vi "Begin.vi"(8 "error in":errorcluster) -> (0 "error out":errorcluster)   [LabVIEW 2020]
doc: "Called before other user functions, this VI is expected to open initial I/O refnums, load in file data, and do all program initialization. Notice that the <B>error out</B> terminal is simply used for data flow. Wiring it to other structures or subVIs ensures that this VI runs first."
uses:
  <vilib>/Rock Robotics/WPI/SafetyOutput/WPI_SafetyOutputConfigMenu.ctl
  <vilib>/Rock Robotics/WPI/DriverStation/WPI_DriverStationRobotMode2.ctl
  <vilib>/Rock Robotics/WPI/Joystick/WPI_JoystickDeviceEnum.ctl
  <vilib>/Rock Robotics/WPI/Solenoid/WPI_SolenoidChannel.ctl
  <vilib>/Rock Robotics/WPI/ThirdParty/REV Robotics/REVLib/Typedef/Spark MAX Idle Mode.ctl
  <vilib>/Rock Robotics/WPI/ThirdParty/Phoenix-LabVIEW/Motor Controller/Controls/CTRE_Phoenix_MotorControl_NeutralMode.ctl
  Robot Global Data.vi
  <vilib>/Rock Robotics/Network Tables/NT Write String Array.vi
  <vilib>/Rock Robotics/WPI/Solenoid/WPI_SolenoidOpenDouble.vi
  <vilib>/Rock Robotics/WPI/RobotDrive/WPI_RobotDriveOpen2MotorWithExistingMotors.vi
  <vilib>/Rock Robotics/WPI/Utilities/WPI_GetSetVariantRefNum.vi
  <vilib>/Rock Robotics/SystemInterfaces/AI/FPGA_AIChannel.ctl
  <vilib>/Rock Robotics/SystemInterfaces/DIO/FPGA_DIOChannel.ctl
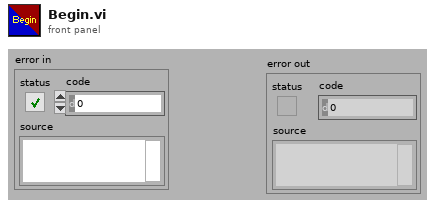
[diagram p1: front panel]
types:
  T1 = typedef "FPGA_DIOChannel.ctl" = enum8{"DIO 0", "DIO 1", "DIO 2", "DIO 3", "DIO 4", "DIO 5", "DIO 6", "DIO 7", "DIO 8", "DIO 9", "DIO MXP 0", "DIO MXP 1", "DIO MXP 2", "DIO MXP 3", "DIO MXP 4", "DIO MXP 5", "DIO MXP 6", "DIO MXP 7", "DIO MXP 8", "DIO MXP 9", "DIO MXP 10", "DIO MXP 11", "DIO MXP 12", "DIO MXP 13", "DIO MXP 14", "DIO MXP 15", "SPI Port CS1", "SPI Port CS2", "SPI Port CS3", "SPI Port MISO", "SPI Port MOSI", "Invalid"}
  T2 = typedef "FPGA_AIChannel.ctl" = enum8{"AI 0", "AI 1", "AI 2", "AI 3", "AI MXP 0", "AI MXP 1", "AI MXP 2", "AI MXP 3", "Invalid"}
  T3 = typedef "Spark MAX Idle Mode.ctl" = enum16{"Coast", "Brake"}
  T4 = typedef "CTRE_Phoenix_MotorControl_NeutralMode.ctl" = enum8{"EEPROMSetting", "Override to Coast", "Override to Brake"}
  T5 = typedef "WPI_SolenoidChannel.ctl" = enum8{"Solenoid 0", "Solenoid 1", "Solenoid 2", "Solenoid 3", "Solenoid 4", "Solenoid 5", "Solenoid 6", "Solenoid 7", "Solenoid 8", "Solenoid 9", "Solenoid 10", "Solenoid 11", "Solenoid 12", "Solenoid 13", "Solenoid 14", "Solenoid 15", "Invalid"}
  T6 = typedef "WPI_JoystickDeviceEnum.ctl" = enum16{"USB 0", "USB 1", "USB 2", "USB 3", "USB 4", "USB 5"}
  T7 = typedef "WPI_DriverStationRobotMode2.ctl" = enum16{"Autonomous Disabled", "Autonomous Enabled", "Teleop Disabled", "Teleop Enabled", "Disconnected", "Finish", "Test Disabled", "Test Enabled", "Emergency Stopped"}
  T8 = typedef "WPI_SafetyOutputConfigMenu.ctl" = enum16{"Enable", "Disable"}
  T9 = typedef "WPI_MotorControlDeviceRef.ctl" = cluster{"DeviceStatus":errorcluster, "Type":T10, "PWM":cluster{"PWM Channel":T11, "DeadBand":T12}, "CAN":cluster{"Device Number":u8, "SetOutput VI Ref":variant, "GetOutput VI Ref":variant, "Enable VI Ref":variant, "Disable VI Ref":variant, "Data":variant}, "Invert":bool, "DIO PWM":cluster{"PWM \"Enable\" Channel":T11, "DIOChannel":T1, "PWM Rate":dbl}}
  T10 = typedef "WPI_MotorControlType.ctl" = enum16{"PWM", "CAN", "DIO PWM"}
  T11 = typedef "FPGA_DIOPWMChannel.ctl" = enum8{"PWM 0", "PWM 1", "PWM 2", "PWM 3", "PWM 4", "PWM 5", "PWM 6", "PWM 7", "PWM 8", "PWM 9", "PWM MXP 0", "PWM MXP 1", "PWM MXP 2", "PWM MXP 3", "PWM MXP 4", "PWM MXP 5", "PWM MXP 6", "PWM MXP 7", "PWM MXP 8", "PWM MXP 9", "Invalid"}
  T12 = typedef "WPI_PWMDeadband.ctl" = cluster{"Name":string, "maxPositivePwm":i32, "minPositivePwm":i32, "centerPwm":i32, "maxNegativePwm":i32, "minNegativePwm":i32, "angularRange":u16}
  T13 = typedef "WPI_JoystickDevRef.ctl" = cluster{"Device":T6}
  T14 = typedef "WPI_RobotDriveDevRef.ctl" = cluster{"DevStatus":errorcluster, "Motors[]":T9[], "Square Inputs":bool, "Max Output":dbl}
  T15 = typedef "CTRE_CANifier_DeviceRef.ctl" = cluster{"DeviceStatus":errorcluster, "Device Number":u8, "Handle":u64, "UsageFrame":u32, "Library Path":path}
  T16 = typedef "WPI_AnalogChannelDevRef.ctl" = cluster{"DevStatus":errorcluster, "Analog Channel":T2}
  T17 = typedef "WPI_DigitalInputDevRef.ctl" = cluster{"DevStatus":errorcluster, "DIO Channel":T1}
  T18 = typedef "WPI_SolenoidDevRef.ctl" = cluster{"DevStatus":errorcluster, "Pneumatics Control Module":u8, "Forward Solenoid Channel":T5, "Reverse Solenoid Channel":T5}
  T19 = typedef "WPI_CompressorDevRef.ctl" = cluster{"DevStatus":errorcluster, "Pneumatics Control Module":u8}
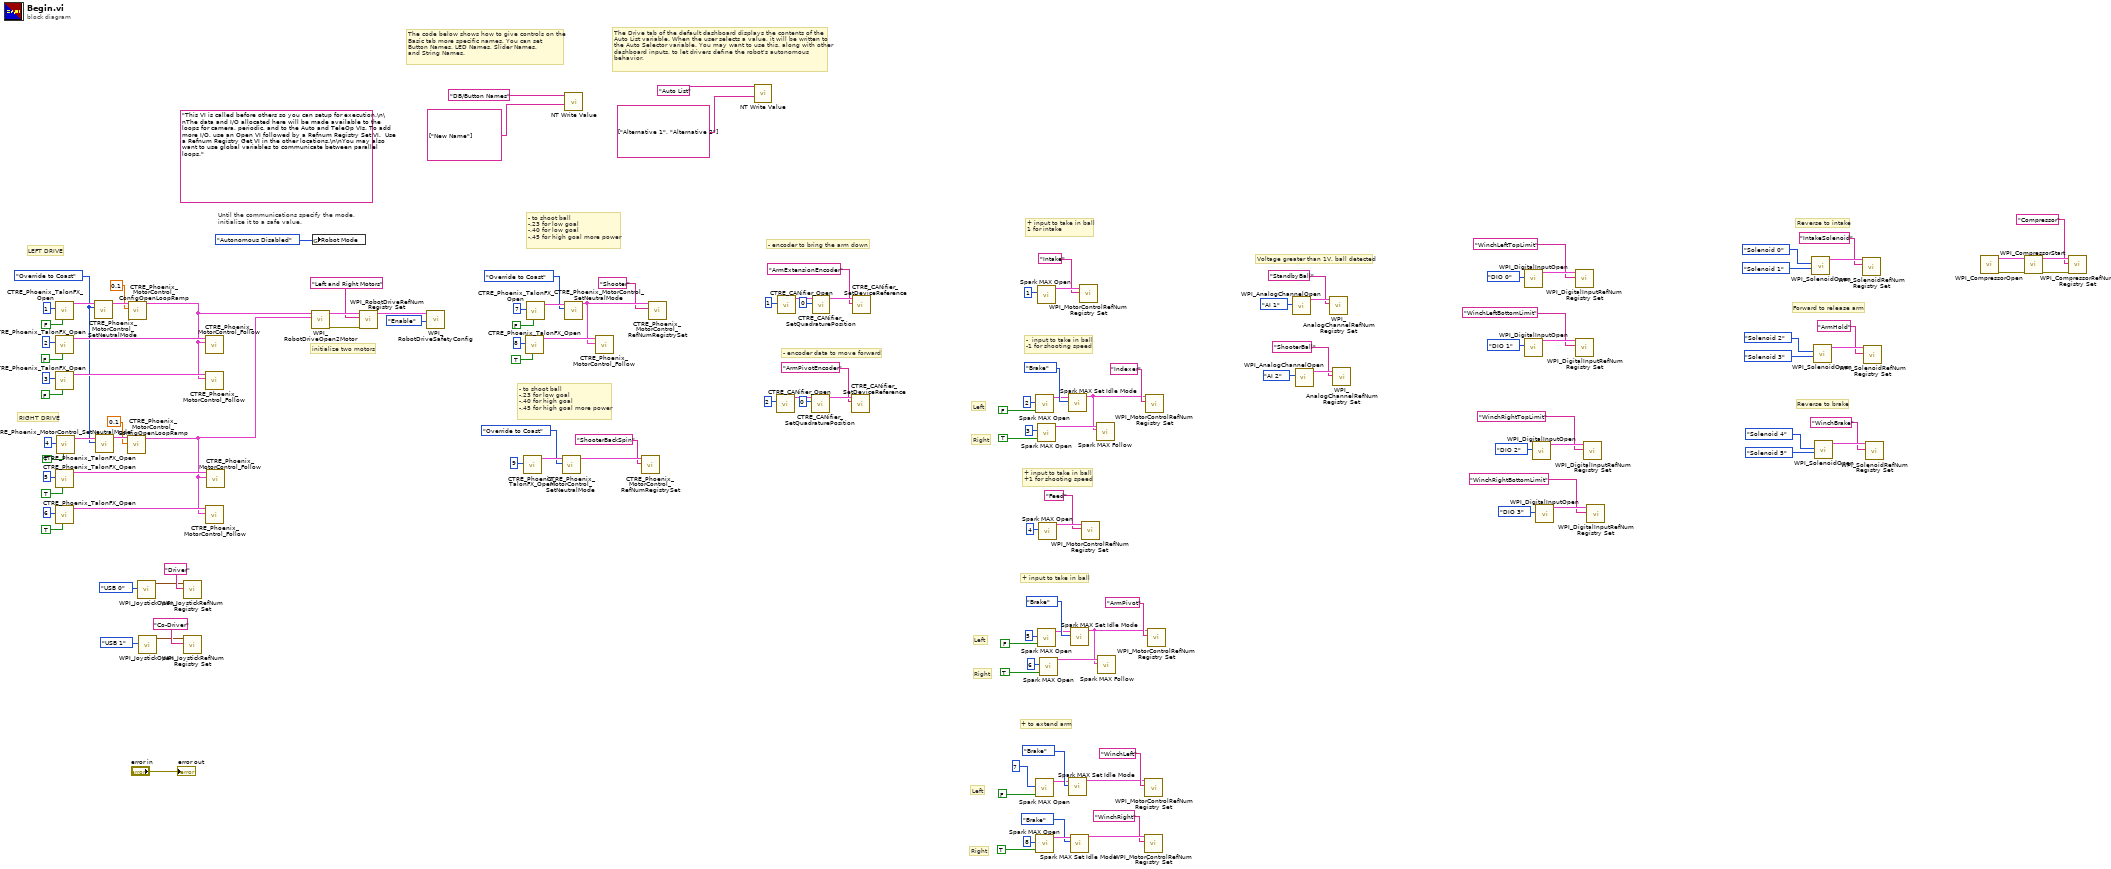
[diagram p0: block diagram]
diagram:
  w100 = CTRE_Phoenix_MotorControl_NeutralMode."Override to Coast" ("Motor Control Neutral Mode")
  (unwired) "This VI is called before others so you can setup for execution.\n\nThe data and I/O allocated here will be made available to the loops for camera, periodic, and to the Auto and TeleOp VIs. To add more I/O, use an Open VI followed by a Refnum Registry Set VI.  Use a Refnum Registry Get VI in the other locations.\n\nYou may also want to use global variables to communicate between parallel loops."
  # "Voltage greater than 1V, ball detected"
  # "- encoder to bring the arm down"
  # "- encoder data to move forward"
  # "- to shoot ball\n-.23 for low goal\n-.40 for high goal\n-.45 for high goal more power"
  # "- to shoot ball\n-.23 for low goal\n-.40 for low goal\n-.45 for high goal more power"
  # "+ to extend arm"
  # "+ input to take in ball"
  # "+ input to take in ball\n+1 for shooting speed"
  # "-  input to take in ball\n-1 for shooting speed"
  # "+ input to take in ball\n1 for intake"
  # "Reverse to brake"
  # "Forward to release arm"
  # "Reverse to intake"
  # "Right"
  # "Left"
  # "Right"
  # "Left"
  # "Right"
  # "Left"
  # "RIGHT DRIVE"
  # "LEFT DRIVE"
  # "The Drive tab of the default dashboard displays the contents of the\nAuto List variable. When the user selects a value, it will be written to\nthe Auto Selector variable. You may want to use this, along with other\ndashboard inputs, to let drivers define the robot's autonomous\nbehavior."
  # "The code below shows how to give controls on the\nBasic tab more specific names. You can set\nButton Names, LED Names, Slider Names,\nand String Names."
  # "Until the communications specify the mode,\ninitialize it to a safe value."
  # "initialize two motors"
  n1 = call <vilib>:"CTRE_Phoenix_TalonFX_Open.vi"("Invert"=FALSE, "Device Number"=u8 2) -> ("PhoenixMotorControlDevRef"=w108:T9)  [unwired: 8 in, 1 out]
  n2 = call <vilib>:"CTRE_Phoenix_TalonFX_Open.vi"("Invert"=FALSE, "Device Number"=u8 3) -> ("PhoenixMotorControlDevRef"=w107:T9)  [unwired: 8 in, 1 out]
  n3 = call <vilib>:"CTRE_Phoenix_TalonFX_Open.vi"("Invert"=FALSE, "Device Number"=u8 1) -> ("PhoenixMotorControlDevRef"=w112:T9)  [unwired: 8 in, 1 out]
  n4 = call <vilib>:"CTRE_Phoenix_TalonFX_Open.vi"("Invert"=TRUE, "Device Number"=u8 5) -> ("PhoenixMotorControlDevRef"=w102:T9)  [unwired: 8 in, 1 out]
  n5 = call <vilib>:"CTRE_Phoenix_TalonFX_Open.vi"("Invert"=TRUE, "Device Number"=u8 6) -> ("PhoenixMotorControlDevRef"=w101:T9)  [unwired: 8 in, 1 out]
  n6 = call <vilib>:"CTRE_Phoenix_TalonFX_Open.vi"("Invert"=TRUE, "Device Number"=u8 4) -> ("PhoenixMotorControlDevRef"=w106:T9)  [unwired: 8 in, 1 out]
  n7 = call <vilib>:"CTRE_Phoenix_MotorControl_SetNeutralMode.vi"("Motor Control Neutral Mode"=w100, "PhoenixMotorControlDevRef"=w112) -> ("PhoenixMotorControlDevRef"=w28:T9)  [unwired: 8 in, 1 out]
  n8 = call <vilib>:"CTRE_Phoenix_MotorControl_SetNeutralMode.vi"("Motor Control Neutral Mode"=w100, "PhoenixMotorControlDevRef"=w106) -> ("PhoenixMotorControlDevRef"=w25:T9)  [unwired: 8 in, 1 out]
  n9 = call <vilib>:"CTRE_Phoenix_MotorControl_ConfigOpenLoopRamp.vi"("secondsFromNeutralToFull"=0.1, "PhoenixMotorControlDevRef"=w25) -> ("PhoenixMotorControlDevRef"=w24:T9)  [unwired: 8 in, 1 out]
  n10 = call <vilib>:"CTRE_Phoenix_MotorControl_ConfigOpenLoopRamp.vi"("secondsFromNeutralToFull"=0.1, "PhoenixMotorControlDevRef"=w28) -> ("PhoenixMotorControlDevRef"=w27:T9)  [unwired: 8 in, 1 out]
  n11 = call <vilib>:"WPI_JoystickOpen.vi"("JoystickDevice"=WPI_JoystickDeviceEnum."USB 0") -> ("JoystickDevRef"=w130:T13)  [unwired: 10 in]
  n12 = call <vilib>:"WPI_JoystickOpen.vi"("JoystickDevice"=WPI_JoystickDeviceEnum."USB 1") -> ("JoystickDevRef"=w114:T13)  [unwired: 10 in]
  n13 = call <vilib>:"WPI_JoystickRefNum Registry Set.vi"("refnum name"="Driver", "JoystickDevRef"=w130) -> ()  [unwired: 8 in, 2 out]
  n14 = call <vilib>:"WPI_JoystickRefNum Registry Set.vi"("refnum name"="Co-Driver", "JoystickDevRef"=w114) -> ()  [unwired: 8 in, 2 out]
  n15 = call <vilib>:"CTRE_Phoenix_MotorControl_Follow.vi"("Master Controller to Follow"=w27, "PhoenixMotorControlDevRef"=w107) -> ()  [unwired: 8 in, 2 out]
  n16 = call <vilib>:"CTRE_Phoenix_MotorControl_Follow.vi"("Master Controller to Follow"=w27, "PhoenixMotorControlDevRef"=w108) -> ()  [unwired: 8 in, 2 out]
  n17 = call <vilib>:"CTRE_Phoenix_MotorControl_Follow.vi"("Master Controller to Follow"=w24, "PhoenixMotorControlDevRef"=w101) -> ()  [unwired: 8 in, 2 out]
  n18 = call <vilib>:"CTRE_Phoenix_MotorControl_Follow.vi"("Master Controller to Follow"=w24, "PhoenixMotorControlDevRef"=w102) -> ()  [unwired: 8 in, 2 out]
  n19 = call-poly <vilib>:"WPI_RobotDriveOpen2Motor.vi"("Right Motor Dev Ref"=w24, "Left Motor Dev Ref"=w27) -> ("error out"=w135:errorcluster, "RobotDriveDevRef"=w137:T14)  [unwired: 3 in, 5 out]
  n20 = global write "Robot Global Data.vi" "Robot Mode"(WPI_DriverStationRobotMode2."Autonomous Disabled" ("Robot Mode")) -> ()
  n21 = call <vilib>:"WPI_RobotDriveRefNum Registry Set.vi"("error in (no error)"=w135, "refnum name"="Left and Right Motors", "RobotDriveDevRef"=w137) -> ("RobotDriveDevRef"=w134:T14)  [unwired: 1 in, 7 out]
  n22 = call <vilib>:"WPI_RobotDriveSafetyConfig.vi"("mode"=WPI_SafetyOutputConfigMenu."Enable", "RobotDriveDevRef"=w134) -> ()  [unwired: 8 in, 2 out]
  n23 = call <vilib>:"CTRE_Phoenix_TalonFX_Open.vi"("Device Number"=u8 9) -> ("PhoenixMotorControlDevRef"=w49:T9)  [unwired: 9 in, 1 out]
  n24 = call <vilib>:"CTRE_Phoenix_TalonFX_Open.vi"("Invert"=TRUE, "Device Number"=u8 8) -> ("PhoenixMotorControlDevRef"=w55:T9)  [unwired: 8 in, 1 out]
  n25 = call <vilib>:"CTRE_Phoenix_TalonFX_Open.vi"("Invert"=FALSE, "Device Number"=u8 7) -> ("PhoenixMotorControlDevRef"=w58:T9)  [unwired: 8 in, 1 out]
  n26 = call <vilib>:"CTRE_Phoenix_MotorControl_SetNeutralMode.vi"("Motor Control Neutral Mode"=CTRE_Phoenix_MotorControl_NeutralMode."Override to Coast", "PhoenixMotorControlDevRef"=w49) -> ("PhoenixMotorControlDevRef"=w46:T9)  [unwired: 8 in, 1 out]
  n27 = call-poly <vilib>:"NT Write Value.vi"("String Array"=string[] ["New Name"], "Name"="DB/Button Names") -> ()  [unwired: 9 in, 1 out]
  n28 = call <vilib>:"CTRE_Phoenix_MotorControl_SetNeutralMode.vi"("Motor Control Neutral Mode"=CTRE_Phoenix_MotorControl_NeutralMode."Override to Coast", "PhoenixMotorControlDevRef"=w58) -> ("PhoenixMotorControlDevRef"=w51:T9)  [unwired: 8 in, 1 out]
  n29 = call <vilib>:"CTRE_Phoenix_MotorControl_Follow.vi"("Master Controller to Follow"=w51, "PhoenixMotorControlDevRef"=w55) -> ()  [unwired: 8 in, 2 out]
  n30 = call <vilib>:"CTRE_Phoenix_MotorControl_RefNumRegistrySet.vi"("refnum name"="ShooterBackSpin", "PhoenixMotorControlDevRef"=w46) -> ()  [unwired: 8 in, 2 out]
  n31 = call <vilib>:"CTRE_Phoenix_MotorControl_RefNumRegistrySet.vi"("refnum name"="Shooter", "PhoenixMotorControlDevRef"=w51) -> ()  [unwired: 8 in, 2 out]
  n32 = call-poly <vilib>:"NT Write Value.vi"("String Array"=string[] ["Alternative 1", "Alternative 2"], "Name"="Auto List") -> ()  [unwired: 9 in, 1 out]
  n33 = call <vilib>:"CTRE_CANifier_Open.vi"("Device Number"=u8 2) -> ("CANifierDevRef"=w38:T15)  [unwired: 9 in, 1 out]
  n34 = call <vilib>:"CTRE_CANifier_Open.vi"("Device Number"=u8 1) -> ("CANifierDevRef"=w43:T15)  [unwired: 9 in, 1 out]
  n35 = call <vilib>:"CTRE_CANifier_SetQuadraturePosition.vi"("newPosition"=0, "CANifierDevRef"=w38) -> ("CANifierDevRef"=w37:T15)  [unwired: 8 in, 1 out]
  n36 = call <vilib>:"CTRE_CANifier_SetQuadraturePosition.vi"("newPosition"=0, "CANifierDevRef"=w43) -> ("CANifierDevRef"=w42:T15)  [unwired: 8 in, 1 out]
  n37 = call <vilib>:"CTRE_CANifier_SetDeviceReference.vi"("refnum name"="ArmPivotEncoder", "CANifierDevRef"=w37) -> ()  [unwired: 8 in, 2 out]
  n38 = call <vilib>:"CTRE_CANifier_SetDeviceReference.vi"("refnum name"="ArmExtensionEncoder", "CANifierDevRef"=w42) -> ()  [unwired: 8 in, 2 out]
  n39 = call <vilib>:"Spark MAX Open.vi"("Invert"=FALSE, "Device Number"=u8 7) -> ("MotorControlDeviceRef"=w63:T9)  [unwired: 8 in, 1 out]
  n40 = call <vilib>:"Spark MAX Open.vi"("Invert"=FALSE, "Device Number"=u8 2) -> ("MotorControlDeviceRef"=w81:T9)  [unwired: 8 in, 1 out]
  n41 = call <vilib>:"Spark MAX Open.vi"("Invert"=TRUE, "Device Number"=u8 8) -> ("MotorControlDeviceRef"=w22:T9)  [unwired: 8 in, 1 out]
  n42 = call <vilib>:"Spark MAX Open.vi"("Device Number"=u8 1) -> ("MotorControlDeviceRef"=w123:T9)  [unwired: 9 in, 1 out]
  n43 = call <vilib>:"Spark MAX Open.vi"("Invert"=TRUE, "Device Number"=u8 3) -> ("MotorControlDeviceRef"=w77:T9)  [unwired: 8 in, 1 out]
  n44 = call <vilib>:"Spark MAX Open.vi"("Invert"=FALSE, "Device Number"=u8 5) -> ("MotorControlDeviceRef"=w72:T9)  [unwired: 8 in, 1 out]
  n45 = call <vilib>:"Spark MAX Open.vi"("Device Number"=u8 4) -> ("MotorControlDeviceRef"=w118:T9)  [unwired: 9 in, 1 out]
  n46 = call <vilib>:"Spark MAX Open.vi"("Invert"=TRUE, "Device Number"=u8 6) -> ("MotorControlDeviceRef"=w68:T9)  [unwired: 8 in, 1 out]
  n47 = call <vilib>:"Spark MAX Set Idle Mode.vi"("Idle Mode"=Spark_MAX_Idle_Mode."Brake", "MotorControlDeviceRef in"=w63) -> ("MotorControlDeviceRef out"=w59:T9)  [unwired: 8 in, 1 out]
  n48 = call <vilib>:"Spark MAX Set Idle Mode.vi"("Idle Mode"=Spark_MAX_Idle_Mode."Brake", "MotorControlDeviceRef in"=w81) -> ("MotorControlDeviceRef out"=w76:T9)  [unwired: 8 in, 1 out]
  n49 = call <vilib>:"Spark MAX Set Idle Mode.vi"("Idle Mode"=Spark_MAX_Idle_Mode."Brake", "MotorControlDeviceRef in"=w22) -> ("MotorControlDeviceRef out"=w20:T9)  [unwired: 8 in, 1 out]
  n50 = call <vilib>:"Spark MAX Set Idle Mode.vi"("Idle Mode"=Spark_MAX_Idle_Mode."Brake", "MotorControlDeviceRef in"=w72) -> ("MotorControlDeviceRef out"=w67:T9)  [unwired: 8 in, 1 out]
  n51 = call <vilib>:"WPI_MotorControlRefNum Registry Set.vi"("refnum name"="Intake", "MotorControlDevRef"=w123) -> ()  [unwired: 8 in, 2 out]
  n52 = call <vilib>:"WPI_MotorControlRefNum Registry Set.vi"("refnum name"="Feed", "MotorControlDevRef"=w118) -> ()  [unwired: 8 in, 2 out]
  n53 = call <vilib>:"Spark MAX Follow.vi"("Master Controller"=w76, "MotorControlDeviceRef"=w77) -> ()  [unwired: 8 in, 2 out]
  n54 = call <vilib>:"Spark MAX Follow.vi"("Master Controller"=w67, "MotorControlDeviceRef"=w68) -> ()  [unwired: 8 in, 2 out]
  n55 = call <vilib>:"WPI_MotorControlRefNum Registry Set.vi"("refnum name"="WinchRight", "MotorControlDevRef"=w20) -> ()  [unwired: 8 in, 2 out]
  n56 = call <vilib>:"WPI_MotorControlRefNum Registry Set.vi"("refnum name"="WinchLeft", "MotorControlDevRef"=w59) -> ()  [unwired: 8 in, 2 out]
  n57 = call <vilib>:"WPI_MotorControlRefNum Registry Set.vi"("refnum name"="Indexer", "MotorControlDevRef"=w76) -> ()  [unwired: 8 in, 2 out]
  n58 = call <vilib>:"WPI_MotorControlRefNum Registry Set.vi"("refnum name"="ArmPivot", "MotorControlDevRef"=w67) -> ()  [unwired: 8 in, 2 out]
  n59 = call <vilib>:"WPI_AnalogChannelOpen.vi"("Analog Channel"=FPGA_AIChannel."AI 1") -> ("AIDeviceRef"=w17:T16)  [unwired: 9 in, 1 out]
  n60 = call <vilib>:"WPI_AnalogChannelOpen.vi"("Analog Channel"=FPGA_AIChannel."AI 2") -> ("AIDeviceRef"=w14:T16)  [unwired: 9 in, 1 out]
  n61 = call <vilib>:"WPI_AnalogChannelRefNum Registry Set.vi"("refnum name"="StandbyBall", "AIDeviceRef"=w17) -> ()  [unwired: 8 in, 2 out]
  n62 = call <vilib>:"WPI_AnalogChannelRefNum Registry Set.vi"("refnum name"="ShooterBall", "AIDeviceRef"=w14) -> ()  [unwired: 8 in, 2 out]
  n63 = call <vilib>:"WPI_DigitalInputOpen.vi"("DIO Channel"=FPGA_DIOChannel."DIO 0") -> ("DigitalInputDevRef"=w12:T17)  [unwired: 9 in, 1 out]
  n64 = call <vilib>:"WPI_DigitalInputOpen.vi"("DIO Channel"=FPGA_DIOChannel."DIO 1") -> ("DigitalInputDevRef"=w6:T17)  [unwired: 9 in, 1 out]
  n65 = call <vilib>:"WPI_DigitalInputOpen.vi"("DIO Channel"=FPGA_DIOChannel."DIO 2") -> ("DigitalInputDevRef"=w9:T17)  [unwired: 9 in, 1 out]
  n66 = call <vilib>:"WPI_DigitalInputOpen.vi"("DIO Channel"=FPGA_DIOChannel."DIO 3") -> ("DigitalInputDevRef"=w3:T17)  [unwired: 9 in, 1 out]
  n67 = call <vilib>:"WPI_DigitalInputRefNum Registry Set.vi"("refnum name"="WinchLeftTopLimit", "DigitalInputDevRef"=w12) -> ()  [unwired: 8 in, 2 out]
  n68 = call <vilib>:"WPI_DigitalInputRefNum Registry Set.vi"("refnum name"="WinchLeftBottomLimit", "DigitalInputDevRef"=w6) -> ()  [unwired: 8 in, 2 out]
  n69 = call <vilib>:"WPI_DigitalInputRefNum Registry Set.vi"("refnum name"="WinchRightTopLimit", "DigitalInputDevRef"=w9) -> ()  [unwired: 8 in, 2 out]
  n70 = call <vilib>:"WPI_DigitalInputRefNum Registry Set.vi"("refnum name"="WinchRightBottomLimit", "DigitalInputDevRef"=w3) -> ()  [unwired: 8 in, 2 out]
  n71 = call-poly <vilib>:"WPI_SolenoidOpen.vi"("Reverse Solenoid Channel"=WPI_SolenoidChannel."Solenoid 1", "Forward Solenoid Channel"=WPI_SolenoidChannel."Solenoid 0") -> ("SolenoidDevRef"=w94:T18)  [unwired: 8 in, 1 out]
  n72 = call-poly <vilib>:"WPI_SolenoidOpen.vi"("Reverse Solenoid Channel"=WPI_SolenoidChannel."Solenoid 3", "Forward Solenoid Channel"=WPI_SolenoidChannel."Solenoid 2") -> ("SolenoidDevRef"=w86:T18)  [unwired: 8 in, 1 out]
  n73 = call-poly <vilib>:"WPI_SolenoidOpen.vi"("Reverse Solenoid Channel"=WPI_SolenoidChannel."Solenoid 5", "Forward Solenoid Channel"=WPI_SolenoidChannel."Solenoid 4") -> ("SolenoidDevRef"=w90:T18)  [unwired: 8 in, 1 out]
  n74 = call <vilib>:"WPI_SolenoidRefNum Registry Set.vi"("refnum name"="IntakeSolenoid", "SolenoidDevRef"=w94) -> ()  [unwired: 8 in, 2 out]
  n75 = call <vilib>:"WPI_SolenoidRefNum Registry Set.vi"("refnum name"="ArmHold", "SolenoidDevRef"=w86) -> ()  [unwired: 8 in, 2 out]
  n76 = call <vilib>:"WPI_SolenoidRefNum Registry Set.vi"("refnum name"="WinchBrake", "SolenoidDevRef"=w90) -> ()  [unwired: 8 in, 2 out]
  n77 = call <vilib>:"WPI_CompressorOpen.vi"() -> ("CompressorDevRef"=w99:T19, "error out"=w96:errorcluster)  [unwired: 14 in]
  n78 = call <vilib>:"WPI_CompressorStart.vi"("error in (no error)"=w96, "CompressorDevRef"=w99) -> ("error out"=w95:errorcluster, "CompressorDevRef"=w98:T19)  [unwired: 8 in]
  n79 = call <vilib>:"WPI_CompressorRefNum Registry Set.vi"("error in (no error)"=w95, "refnum name"="Compressor", "CompressorDevRef"=w98) -> ()  [unwired: 7 in, 2 out]
  "error out" <- "error in"
